vi "I2C Get Num Channels.vi"(8 "error in (no error)":errorcluster) -> (0 "error out":errorcluster, 3 "numChannels":u32)   [LabVIEW 2024, in "libMPSSE-I2C.lvlib"]
doc: "FTDI_API FT_STATUS SPI_GetNumChannels(uint32 *numChannels);"
uses:
  libMPSSE-I2C.lvlib
  libmpsse.dll
panel:
  out "return type":u32
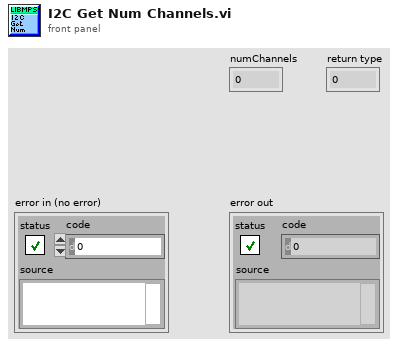
[diagram p1: front panel]
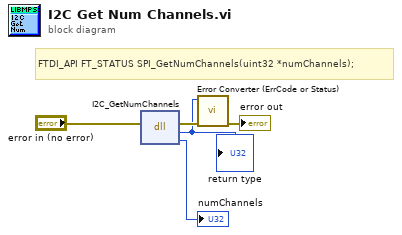
[diagram p0: block diagram]
diagram:
  # "FTDI_API FT_STATUS SPI_GetNumChannels(uint32 *numChannels);"
  n1 = dll-call lib="libmpsse.dll" fn="I2C_GetNumChannels"(error in="error in (no error)") -> (error out=w3:errorcluster, "return type"=w1:u32, "numChannels"=→"numChannels":u32)  [unwired: 3 in, 1 out]
  "return type" <- w1
  n2 = call "Error Converter (ErrCode or Status).vi"("error in (no error)"=w3, "error code"=w1) -> ("error out"=→"error out":errorcluster)  [unwired: 9 in]
